vi "poly_is_poly_vi_ref.vi"(2 "vi ref":refnum<vi>) -> (7 "is poly vi?":bool)   [LabVIEW 2015]
uses:
  <vilib>/Utility/Data Type/Type Definitions/Data Type.ctl
  <vilib>/Utility/Data Type/NI_Data Type.lvlib
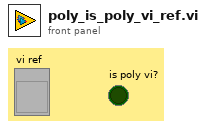
[diagram p1: front panel]
types:
  T1 = typedef "NI_Data Type.lvlib/Data Type.ctl" = enum8{"Invalid Type", "Void", "I8", "I16", "I32", "I64", "U8", "U16", "U32", "U64", "Single Float", "Double Float", "Extended Float", "Single Complex", "Double Complex", "Extended Complex", "Enum U8", "Enum U16", "Enum U32", "Enum U64", "Single Float With Unit", "Double Float With Unit", "Extended Float With Unit", "Single Complex with Unit", "Double Complex with Unit", "Extended Complex with Unit", "Boolean", "String", "Path", "Picture", "Tag", "Array", "Cluster", "Variant", "LV Variant", "Waveform", "Timestamp", "Digital Waveform", "Digital Data", "ExpressData", "Refnum", "External Data", "VI", "Poly VI", "LabVIEW Class Instance", "Fixed Point"}
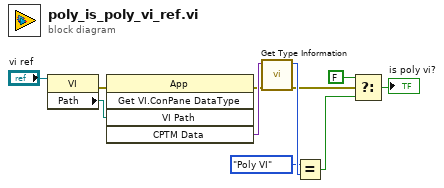
[diagram p0: block diagram]
diagram:
  n1 = property class="VI"(reference="vi ref") -> (error out=w1:errorcluster, "Path"=w3:path)  [unwired: 1 in, 1 out]
  n2 = invoke class="App" method="Get VI.ConPane DataType"(error in=w1, "VI Path"=w3) -> (error out=w10:errorcluster, "CPTM Data"=w11:variant)  [unwired: 3 in, 3 out]
  n3 = call <vilib>:"Get Type Information.vi"("error in (no error)"=w10, "Variant"=w11) -> ("error out"=w7:errorcluster, "Type"=w9:T1)  [unwired: 5 in, 3 out]
  n4 = Equal?(x=Data_Type."Poly VI" ("Type"), y=w9) -> (x = y?=w6:bool)
  n5 = Select(t=FALSE, s=w7, f=w6) -> (s? t:f=→"is poly vi?":bool)
